vi "SUB_Ping_IP_Status.vi"(0 "IP Address":string) -> (1 "ok":bool, 2 "standard output":string)   [LabVIEW 2011]
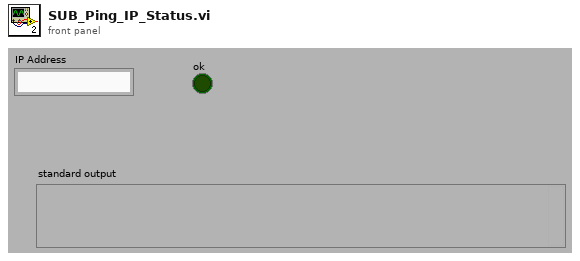
[diagram p1: front panel]
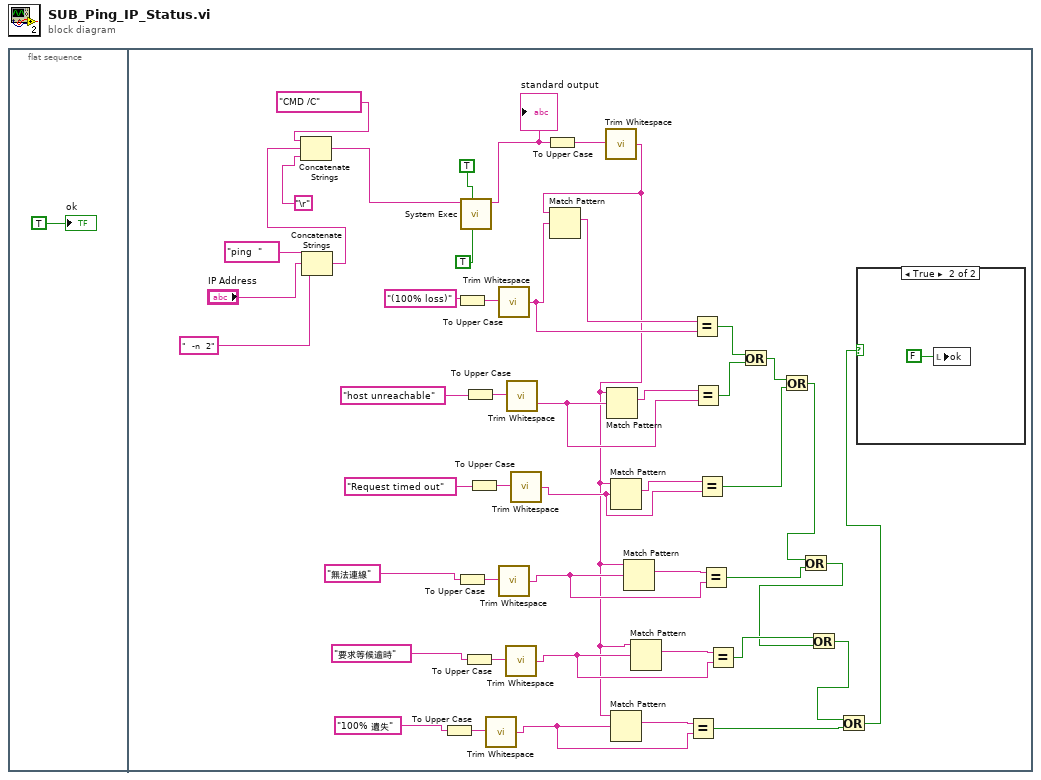
[diagram p0: block diagram]
diagram:
  n1 = flat-sequence {
    frame #0 {
      "ok" <- TRUE ("Found error")
    }
    frame #1 {
      n2 = Concatenate Strings("ping  ", "IP Address", "  -n  2") -> (w42:string)
      n3 = Concatenate Strings("CMD /C", w42, "\r") -> (w45:string)
      n4 = To Upper Case(1:"100% 遺失") -> (0:w9:string)
      n5 = To Upper Case(1:"(100% loss)") -> (0:w37:string)
      n6 = To Upper Case(1:"無法連線") -> (0:w21:string)
      n7 = call <vilib>:"System Exec.vi"("run minimized? (F)"=TRUE, "wait until completion? (T)"=TRUE, "command line"=w45) -> ("standard output"=w38:string)  [unwired: 5 in, 3 out]
      "standard output" <- w38
      n8 = To Upper Case(1:"要求等候逾時") -> (0:w15:string)
      n9 = To Upper Case(1:"host unreachable") -> (0:w34:string)
      n10 = To Upper Case(1:"Request timed out") -> (0:w26:string)
      n11 = call <vilib>:"Trim Whitespace.vi"("string"=w9) -> ("trimmed string"=w8:string)  [unwired: 1 in]
      n12 = call <vilib>:"Trim Whitespace.vi"("string"=w37) -> ("trimmed string"=w35:string)  [unwired: 1 in]
      n13 = call <vilib>:"Trim Whitespace.vi"("string"=w21) -> ("trimmed string"=w19:string)  [unwired: 1 in]
      n14 = call <vilib>:"Trim Whitespace.vi"("string"=w15) -> ("trimmed string"=w13:string)  [unwired: 1 in]
      n15 = call <vilib>:"Trim Whitespace.vi"("string"=w34) -> ("trimmed string"=w31:string)  [unwired: 1 in]
      n16 = call <vilib>:"Trim Whitespace.vi"("string"=w26) -> ("trimmed string"=w23:string)  [unwired: 1 in]
      n17 = To Upper Case(1:w38) -> (0:w39:string)
      n18 = call <vilib>:"Trim Whitespace.vi"("string"=w39) -> ("trimmed string"=w2:string)  [unwired: 1 in]
      n19 = Match Pattern(string=w2, regular expression=w35) -> (match substring=w41:string)  [unwired: 1 in, 3 out]
      n20 = Match Pattern(string=w2, regular expression=w31) -> (match substring=w32:string)  [unwired: 1 in, 3 out]
      n21 = Match Pattern(string=w2, regular expression=w23) -> (match substring=w24:string)  [unwired: 1 in, 3 out]
      n22 = Match Pattern(string=w2, regular expression=w8) -> (match substring=w7:string)  [unwired: 1 in, 3 out]
      n23 = Match Pattern(string=w2, regular expression=w19) -> (match substring=w18:string)  [unwired: 1 in, 3 out]
      n24 = Match Pattern(string=w2, regular expression=w13) -> (match substring=w12:string)  [unwired: 1 in, 3 out]
      n25 = Equal?(x=w7, y=w8) -> (x = y?=w4:bool)
      n26 = Equal?(x=w41, y=w35) -> (x = y?=w30:bool)
      n27 = Equal?(x=w32, y=w31) -> (x = y?=w29:bool)
      n28 = Equal?(x=w24, y=w23) -> (x = y?=w22:bool)
      n29 = Equal?(x=w18, y=w19) -> (x = y?=w16:bool)
      n30 = Equal?(x=w12, y=w13) -> (x = y?=w11:bool)
      n31 = Or(x=w30, y=w29) -> (x .or. y?=w27:bool)
      n32 = Or(x=w27, y=w22) -> (x .or. y?=w17:bool)
      n33 = Or(x=w17, y=w16) -> (x .or. y?=w10:bool)
      n34 = Or(x=w11, y=w10) -> (x .or. y?=w5:bool)
      n35 = Or(x=w5, y=w4) -> (x .or. y?=w3:bool)
      n36 = case shown="True" w3 {
        frame False {
        }
        frame True {
          n37 = local write "ok"(FALSE ("ok")) -> ()
        }
      }
    }
  }
